vi "Check and Reestablish Connection.vi"(9 "CD Path":string, 10 "IP Address":string, 11 "connection info":T1) -> (0 "error out":errorcluster, 3 "connection info":T1)   [LabVIEW 2015, in "J1939 Addon Shared.lvlib"]
uses:
  J1939 Addon Shared.lvlib
  <vilib>/NI/STM/TCP/TCP Connection Info.ctl
  <vilib>/NI/STM/SubVIs/MetaDataElement.ctl
  <vilib>/NI/STM/NI STM.lvlib
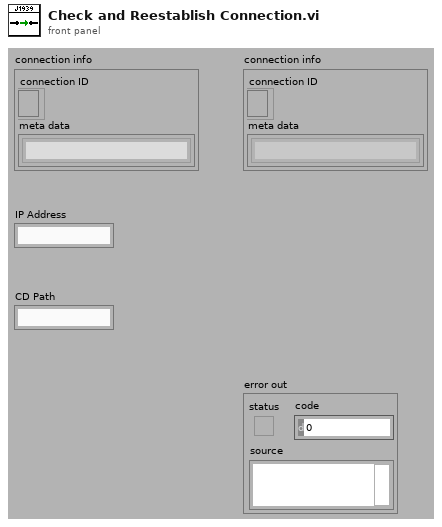
[diagram p1: front panel]
types:
  T1 = typedef "NI STM.lvlib/TCP Connection Info.ctl" = cluster{"connection ID":refnum<k5>, "meta data":T2[]}
  T2 = typedef "NI STM.lvlib/MetaDataElement.ctl" = string
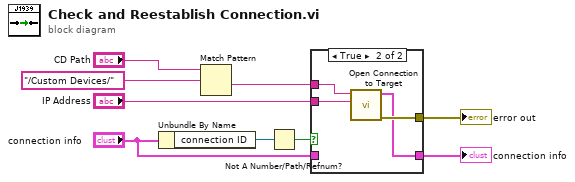
[diagram p0: block diagram]
diagram:
  n1 = Unbundle By Name("connection info") -> ("connection ID"=w4:refnum<k5>)
  n2 = Match Pattern(string="CD Path", regular expression="/Custom Devices/" ("Custom Device Path")) -> (after substring=w1:string)  [unwired: 1 in, 3 out]
  n3 = Not A Number/Path/Refnum?(number/path/refnum=w4) -> (NaN/Path/Refnum?=w8:bool)
  n4 = case shown="True" w8 {
    tunnel: w1 -> [_ w12]
    tunnel: [w10 w13] -> w6
    tunnel: "connection info" -> [w10 _]
    tunnel: [_ w14] -> w9
    tunnel: "IP Address" -> [_ w11]
    frame False {
    }
    frame True {
      n5 = call "Open Connection to Target.vi"("IP Address"=w11, "TCP Service"=w12) -> ("error out"=w14:errorcluster, "connection info"=w13:T1)  [unwired: 8 in]
    }
  }
  "error out" <- w9
  "connection info" <- w6
